vi "MAS_Query.vi"(0 "System no.":i32=1 min=1 max=4 step=1, 2 "Axes to query":string[](array[string]), 3 "All axes?":bool, 4 "Axis identifier?":bool=TRUE, 5 "error in":errorcluster) -> (14 "Master axis":string[](array[string]), 19 "error out":errorcluster)   [LabVIEW 2020]
doc: "Returns the master axis for the specified axis.\n\nC-843, C-848, C-880: If All axes = TRUE, then Axis identifier can be FALSE."
panel:
  # "Returns the master axis for the specified axis."
  # "If all axes: use"
  # "Query"
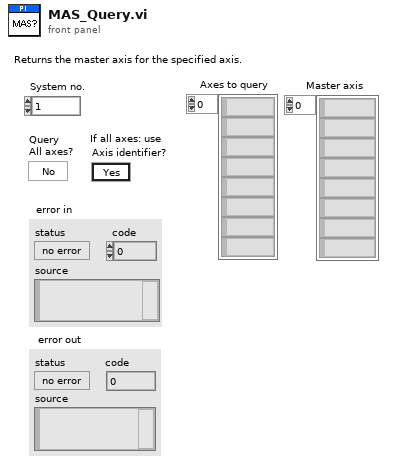
[diagram p1: front panel]
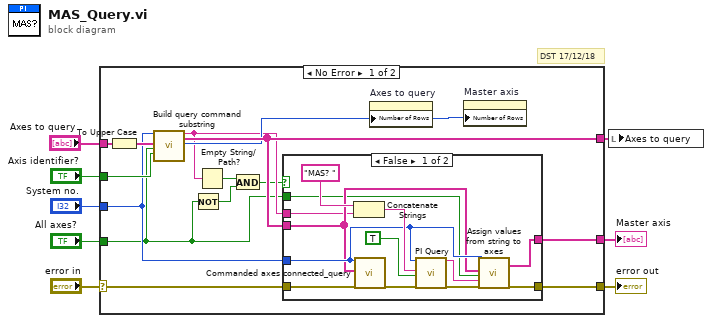
[diagram p0: block diagram]
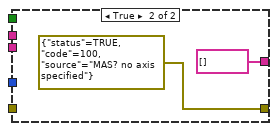
[diagram p2: hidden frame]
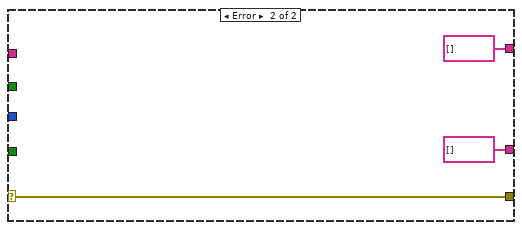
[diagram p3: hidden frame]
diagram:
  # "DST 17/12/18"
  n1 = case shown="No Error" "error in" {
    selector: "error in" -> [w11 w38]
    tunnel: [w15 string[] [] ("Strings")] -> w2
    tunnel: "Axes to query" -> [w22 _]
    tunnel: [w21 w38] -> w7
    tunnel: "Axis identifier?" -> [w19 _]
    tunnel: "System no." -> [w18 _]
    tunnel: [w17 string[] [] ("Axes to query out")] -> w4
    tunnel: "All axes?" -> [w9 _]
    frame No Error {
      n2 = To Upper Case(1:w22) -> (0:w20:string[])
      n3 = call "Build query command substring.vi"("System no."=w18, "Axes to query in"=w20, "Query\nAll axes?"=w9, "For all axes: use\nAxis identifier?"=w19) -> ("Command substring"=w13:string, "Axes to query out"=w17:string[], "Number of rows"=w14:u32)  [unwired: 2 in, 11 out]
      n4 = Not(x=w9) -> (.not. x?=w16:bool)
      n5 = Empty String/Path?(string/path=w13) -> (empty?=w12:bool)
      n6 = And(x=w12, y=w16) -> (x .and. y?=w10:bool)
      n7 = case shown="False" w10 {
        tunnel: [w23 errorcluster {"status"=TRUE, "code"=100, "source"="MAS? no axis specified"} ("error out")] -> w21
        tunnel: w18 -> [w32 _]
        tunnel: w17 -> [w31 _]
        tunnel: w9 -> [w30 _]
        tunnel: [w28 string[] [] ("Strings")] -> w15
        tunnel: w13 -> [w27 _]
        tunnel: w11 -> [w26 _]
        frame False {
          n8 = Concatenate Strings("MAS? ", w27) -> (w33:string)
          n9 = call "Commanded axes connected_query.vi"("System no."=w32, "Commanded axes"=w31, "error in"=w26) -> ("error out"=w29:errorcluster)  [unwired: 1 in, 15 out]
          n10 = call "PI Query.vi"("System no."=w32, "String to send"=w33, "Attach termination char.?"=TRUE ("Attach Linefeed?"), "error in"=w29) -> ("String read"=w25:string, "error out"=w24:errorcluster)  [unwired: 3 in, 11 out]
          n11 = call "Assign values from string to axes.vi"("System no."=w32, "Queried axes"=w31, "All axes queried?"=w30, "Input String"=w25, "error in"=w24) -> ("Strings"=w28:string[], "error out"=w23:errorcluster)  [unwired: 4 in, 9 out]
        }
        frame True {
        }
      }
      n12 = property on="Axes to query" class="Arr (strict)"("Number of Rows"=w14) -> ()  [unwired: 2 in, 2 out]
      n13 = property on="Master axis" class="Arr (strict)"("Number of Rows"=w14) -> ()  [unwired: 2 in, 2 out]
    }
    frame Error {
    }
  }
  "error out" <- w7
  "Master axis" <- w2
  n14 = local write "Axes to query"(w4) -> ()
